vi "2021 Advent puzzle 01.vi"() -> ()   [LabVIEW 2021]
panel:
  out "sum":i16
  out "?":i16[](array[numeric])
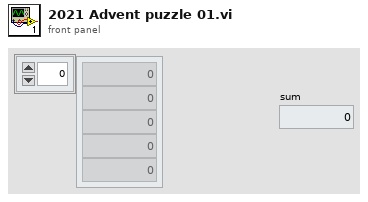
[diagram p1: front panel]
diagram:
  # "find the number of increasing values"
  n1 = Spreadsheet String To Array(delimiter (Tab)="\n", format string="", spreadsheet string="188\n192\n193\n194\n192\n213\n214\n216\n219\n221\n222\n228\n231\n234\n239\n240\n252\n262\n267\n279\n278\n277\n279\n293\n309\n310\n312\n307\n308\n316\n320\n323\n335\n336\n343\n368\n357\n370\n377\n386\n387\n386\n402\n379\n393\n394\n403\n404\n405\n400\n421\n422\n423\n408\n409\n411\n408\n415\n417\n430\n439\n432\n459\n462\n463\n464\n466\n472\n485\n473\n488\n491\n492\n493\n496\n497\n501\n503\n516\n514\n513\n514\n517\n521\n522\n526\n548\n553\n560\n563\n565\n600\n601\n595\n596\n597\n599\n613\n630\n631\n635\n642\n648\n651\n654\n645\n653\n657\n676\n688\n711\n717\n718\n728\n735\n730\n733\n734\n737\n736\n738\n741\n749\n751\n752\n762\n765\n776\n779\n758\n743\n754\n759\n772\n773\n783\n790\n791\n783\n781\n784\n785\n791\n780\n789\n805\n792\n793\n797\n825\n...", array type (2D Dbl)=i32[] []) -> (array=w6:i32[])
  n2 = Delete From Array(array=w6, index=0 ("length")) -> (deleted portion=w4:i32, array with subset deleted=w5:i32[])  [unwired: 1 in]
  n3 = for {
    tunnel: w5 -> [w13] mode=indexing
    shift-right: [w13] -> _
    shift-left: w4 -> [w14]
    tunnel: [w11] -> w2 mode=indexing
    n4 = Greater?(x=w13, y=w14) -> (0:w12:bool)
    n5 = Boolean To (0,1)(Boolean=w12) -> (0, 1=w11:i16)
  }
  "?" <- w2
  n6 = Add Array Elements(numeric array=w2) -> (sum=→"sum":i16)
